vi "getSymbol.vi"(8 "error in (no error)":errorcluster, 11 "IUnit in":refnum<class "IUnit.lvclass">) -> (0 "error out":errorcluster, 2 "Symbol out":string, 3 "IUnit out":refnum<class "IUnit.lvclass">)   [LabVIEW 2022 SP3, in "openDAQ.lvlib" / "IBaseObject.lvlib" / "IUnit.lvlib" / "IUnit.lvclass"]
uses:
  <instrlib>/openDAQ/Public/Classes/IUnit/IUnit.lvclass
  C:/Program Files (x86)/National Instruments/LabVIEW 2022/instr.lib/openDAQ/Public/Classes/IBaseObject/IBaseObject.lvclass
  <instrlib>/openDAQ/Public/Classes/daqCoreTypes/IString/IString.lvclass
  <instrlib>/openDAQ/Public/Classes/IBaseObject/IBaseObject.lvclass/IBaseObject.ctl
  <instrlib>/openDAQ/Public/Classes/IBaseObject/Accessor/Write reference.vi
  <instrlib>/openDAQ/Public/Classes/IBaseObject/Accessor/Read reference.vi
  <instrlib>/openDAQ/Binaries/Windows/x86/copendaq32.dll
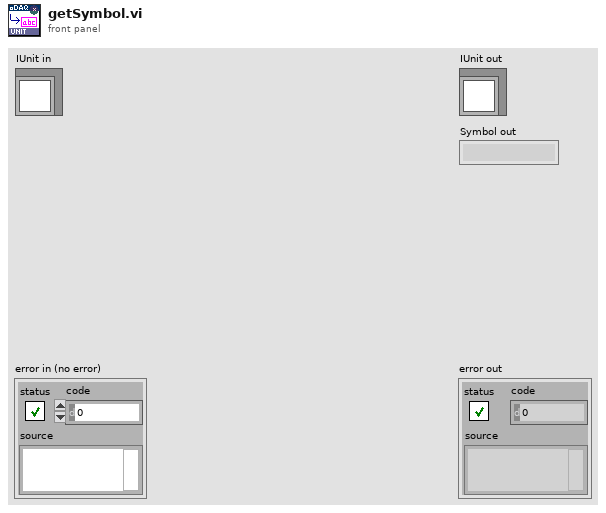
[diagram p1: front panel]
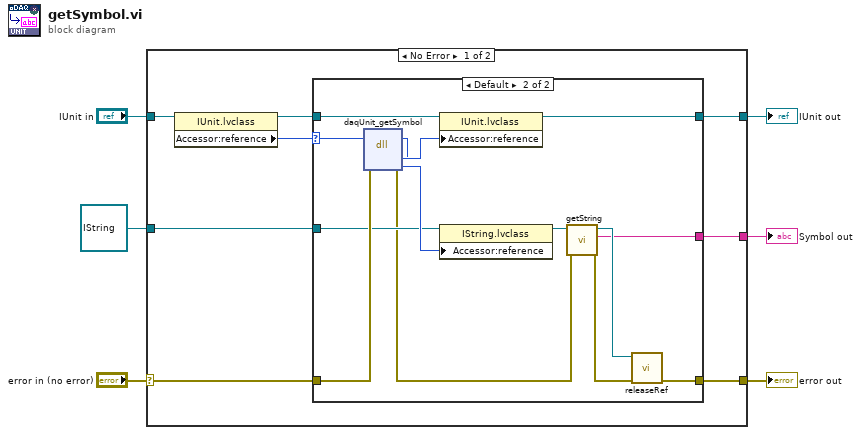
[diagram p0: block diagram]
diagram:
  n1 = case shown="No Error" "error in (no error)" {
    selector: "error in (no error)" -> [w13 w31]
    tunnel: [w9 w31] -> w5
    tunnel: [w11 w30] -> w3
    tunnel: "IUnit in" -> [w14 w30]
    tunnel: refnum<class "IString.lvclass"> refnum ("openDAQ.lvlib:daqCoreTypes.lvlib:IString.lvclass") -> [w10 _]
    tunnel: [w8 _] -> w1
    frame No Error {
      n2 = property class="IUnit.lvclass"(reference=w14) -> (reference out=w12:refnum<class "IUnit.lvclass">, "Accessor:reference"=w7:i64)  [unwired: 1 in, 1 out]
      n3 = case shown="Default" w7 {
        selector: w7 -> [_ w17]
        tunnel: w13 -> [w15 w28]
        tunnel: w12 -> [w16 w27]
        tunnel: [w16 w26] -> w11
        tunnel: w10 -> [_ w24]
        tunnel: [w15 w19] -> w9
        tunnel: [_ w18] -> w8
        frame 0 {
        }
        frame Default {
          n4 = dll-call lib="C:/Program Files (x86)/National Instruments/LabVIEW 2022/instr.lib/openDAQ/Binaries/Windows/x86/copendaq*.*" fn="daqUnit_getSymbol"(error in=w28, "unit"=w17) -> (error out=w22:errorcluster, "unit"=w25:i64, "symbol"=w29:i64)  [unwired: 4 in, 1 out]
          n5 = property class="IUnit.lvclass"(reference=w27, "Accessor:reference"=w25) -> (reference out=w26:refnum<class "IUnit.lvclass">)  [unwired: 1 in, 1 out]
          n6 = property class="IString.lvclass"(reference=w24, "Accessor:reference"=w29) -> (reference out=w23:refnum<class "IString.lvclass">)  [unwired: 1 in, 1 out]
          n7 = call <instrlib>:"getString.vi"("error in (no error)"=w22, "IString in"=w23) -> ("error out"=w20:errorcluster, "String out"=w18:string, "IString out"=w21:refnum<class "IString.lvclass">)  [unwired: 7 in]
          n8 = call-dynamic "releaseRef.vi"("error in (no error)"=w20, "IBaseObject in"=w21) -> ("error out"=w19:errorcluster)  [unwired: 9 in]
        }
      }
    }
    frame Error {
    }
  }
  "error out" <- w5
  "IUnit out" <- w3
  "Symbol out" <- w1
